vi "OP500ZP_FDT.vi"(8 "errin":errorcluster caption="entrée d'erreur (pas d'erreur)") -> (0 "errout":errorcluster caption="sortie d'erreur", 1 "FDT":T1, 3 "True/False":bool)   [LabVIEW 2020]
uses:
  VG/PackType.vi
  VG/IS30%.vi
panel:
  out "DELTA TEMP":bool
  out "TCELL<ref":bool
  out "TCELL>ref":bool
  out "VCELL>ref":bool
  out "VCELL<ref":bool
  out "DELTA V":bool
  out "UBATT":bool
  out "PASS/FAIL?":string
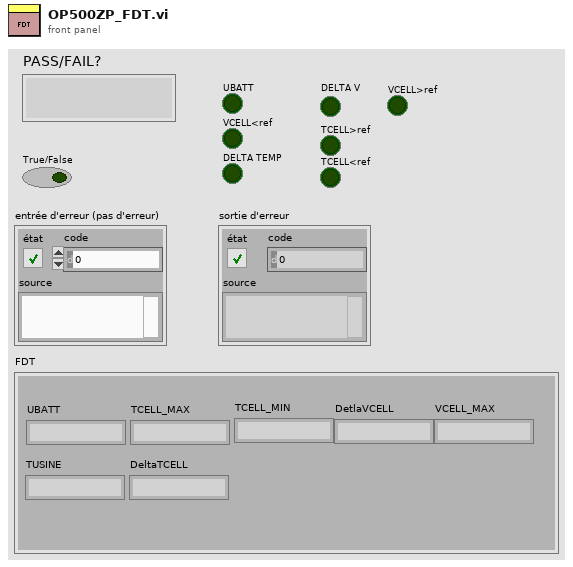
[diagram p1: front panel]
types:
  T1 = cluster{"UBATT":string, "TCELL_MAX":string, "TCELL_MIN":string, "DetlaVCELL":string, "VCELL_MAX":string, "TUSINE":string, "DeltaTCELL":string}
  T2 = cluster{string, string, string, string, string, string, string}
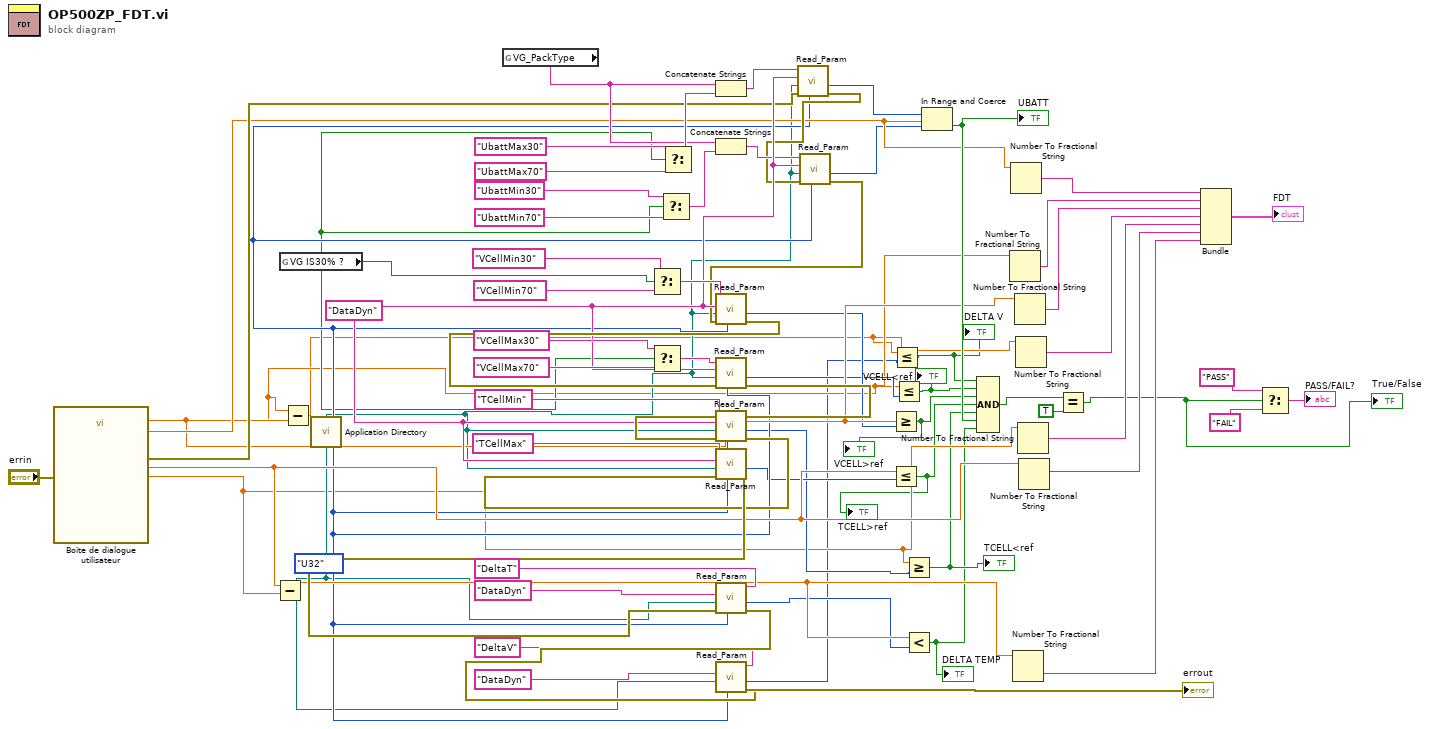
[diagram p0: block diagram]
diagram:
  w24 = enum16{"STR", "DBL", "U32"}."U32" ("Énum")
  w48 = "DataDyn" ("section")
  n1 = call "Boîte de dialogue utilisateur"("error in (no error)"="errin") -> ("Min Cell Temeprature"=w12:dbl, "Max Cell Temperature"=w36:dbl, "Min Cell Voltage"=w37:dbl, "Max Cell Voltage"=w14:dbl, "Battery Voltage"=w38:dbl, "error out"=w41:errorcluster)  [unwired: 11 in, 2 out]
  n2 = Subtract(x=w36, y=w12) -> (x-y=w35:dbl)
  n3 = global read "IS30%.vi" "VG IS30% ?"() -> (w17:bool)
  n4 = Subtract(x=w14, y=w37) -> (x-y=w3:dbl)
  n5 = call <vilib>:"Application Directory.vi"() -> ("Application Directory"=w23:path)
  n6 = global read "PackType.vi" "VG_PackType"() -> (w45:string)
  n7 = Select ("Sélectionner")(t="VCellMin30" ("key"), s=w17, f="VCellMin70" ("key")) -> (s? t:f=w60:string)
  n8 = Select ("Sélectionner")(t="VCellMax30" ("key"), s=w17, f="VCellMax70" ("key")) -> (s? t:f=w61:string)
  n9 = Select ("Sélectionner")(t="UbattMin30", s=w17, f="UbattMin70") -> (s? t:f=w44:string)
  n10 = Select ("Sélectionner")(t="UbattMax30", s=w17, f="UbattMax70" ("cas faux")) -> (s? t:f=w47:string)
  n11 = Concatenate Strings(w45, w47) -> (w46:string)
  n12 = Concatenate Strings(w45, w44) -> (w43:string)
  n13 = call <userlib>:"Read_Param.vi"("Énum"=w24, "errin"=w41, "pathin"=w23, "section"=w48, "key"=w46) -> ("error out"=w40:errorcluster, "U32"=w18:u32)  [unwired: 2 in, 3 out]
  n14 = call <userlib>:"Read_Param.vi"("Énum"=w24, "errin"=w40, "pathin"=w23, "section"=w48, "key"=w43) -> ("error out"=w39:errorcluster, "U32"=w19:u32)  [unwired: 2 in, 3 out]
  n15 = call <userlib>:"Read_Param.vi"("Énum"=w24, "errin"=w39, "pathin"=w23, "section"=w48, "key"=w60) -> ("error out"=w62:errorcluster, "U32"=w20:u32)  [unwired: 2 in, 3 out]
  n16 = call <userlib>:"Read_Param.vi"("Énum"=w24, "errin"=w62, "pathin"=w23, "section"=w48, "key"=w61) -> ("error out"=w63:errorcluster, "U32"=w15:u32)  [unwired: 2 in, 3 out]
  n17 = call <userlib>:"Read_Param.vi"("Énum"=w24, "errin"=w63, "pathin"=w23, "section"=w48, "key"="TCellMin") -> ("error out"=w59:errorcluster, "U32"=w13:u32)  [unwired: 2 in, 3 out]
  n18 = call <userlib>:"Read_Param.vi"("Énum"=w24, "errin"=w59, "pathin"=w23, "section"=w48, "key"="TCellMax") -> ("error out"=w69:errorcluster, "U32"=w21:u32)  [unwired: 2 in, 3 out]
  n19 = call <userlib>:"Read_Param.vi"("Énum"=w24, "errin"=w69, "pathin"=w23, "section"="DataDyn", "key"="DeltaT") -> ("error out"=w70:errorcluster, "U32"=w22:u32)  [unwired: 2 in, 3 out]
  n20 = call <userlib>:"Read_Param.vi"("Énum"=w24, "errin"=w70, "pathin"=w23, "section"="DataDyn", "key"="DeltaV") -> ("error out"=→"errout":errorcluster, "U32"=w2:u32)  [unwired: 2 in, 3 out]
  n21 = Greater Or Equal?(x=w37, y=w20) -> (x >= y?=w7:bool)
  "VCELL>ref" <- w7
  n22 = Less Or Equal?(x=w36, y=w21) -> (x <= y?=w6:bool)
  "TCELL>ref" <- w6
  n23 = Less Or Equal?(x=w3, y=w2) -> (x <= y?=w1:bool)
  "DELTA V" <- w1
  n24 = Less Or Equal?(x=w14, y=w15) -> (x <= y?=w16:bool)
  "VCELL<ref" <- w16
  n25 = Greater Or Equal?(x=w12, y=w13) -> (x >= y?=w5:bool)
  "TCELL<ref" <- w5
  n26 = Less?(x=w35, y=w22) -> (x < y?=w4:bool)
  "DELTA TEMP" <- w4
  n27 = In Range and Coerce(upper limit=w18, x=w38, lower limit=w19) -> (In Range?=w42:bool)  [unwired: 1 out]
  "UBATT" <- w42
  n28 = Compound Arithmetic op=AND ("Opérateur arithmétique")(w1, w16, w7, w6, w5, w42, w4) -> (w26:bool)
  n29 = Number To Fractional String(number=w14) -> (F-format string=w33:string)  [unwired: 3 in]
  n30 = Number To Fractional String(number=w38) -> (F-format string=w34:string)  [unwired: 3 in]
  n31 = Number To Fractional String(number=w35) -> (F-format string=w28:string)  [unwired: 3 in]
  n32 = Number To Fractional String(number=w37) -> (F-format string=w32:string)  [unwired: 3 in]
  n33 = Number To Fractional String(number=w3) -> (F-format string=w31:string)  [unwired: 3 in]
  n34 = Number To Fractional String(number=w12) -> (F-format string=w30:string)  [unwired: 3 in]
  n35 = Number To Fractional String(number=w36) -> (F-format string=w29:string)  [unwired: 3 in]
  n36 = Equal?(x=w26, y=TRUE) -> (x = y?=w9:bool)
  "True/False" <- w9
  n37 = Bundle(w34, w33, w32, w31, w30, w29, w28) -> (→"FDT":T2)  [unwired: 1 in]
  n38 = Select ("Sélectionner")(t="PASS", s=w9, f="FAIL") -> (s? t:f=→"PASS/FAIL?":string)
